vi "disdrometer_output.vi"(0 "Filepath":path, 5 "Data Array":string[](array[string]), 7 "Timestamp":dbl, 9 "Format String":string[](array[string])=["000", "001", "002"], 11 "Error In":errorcluster) -> (15 "Error Out":errorcluster)   [LabVIEW 2018]
doc: "Creates or appends a line to a text file at Filepath, adding the data in Data Array. Appends the Timestamp to the front of the line, and formats the array with tabs between each element."
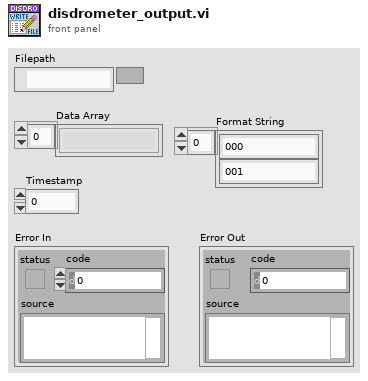
[diagram p1: front panel]
types:
  T1 = enum16{"open", "replace", "create", "open or create", "replace or create", "replace or create with confirmation"}
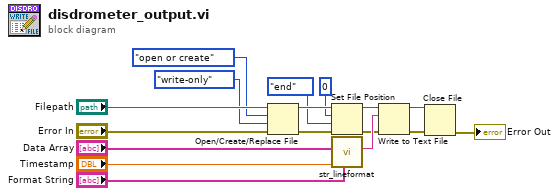
[diagram p0: block diagram]
diagram:
  n1 = Open/Create/Replace File(file path (use dialog)="Filepath", error in="Error In", operation (0:open)=T1."open or create", access (0:read/write)=enum16{"read/write", "read-only", "write-only"}."write-only") -> (refnum out=w11:refnum<file>, error out=w10:errorcluster)  [unwired: 3 out]
  n2 = Set File Position(offset (in bytes) (0)=i64 0, refnum=w11, from (0:start)=enum16{"start", "end", "current"}."end", error in=w10) -> (refnum out=w8:refnum<file>, error out=w9:errorcluster)
  n3 = call "str_lineformat.vi"("Format String"="Format String", "Timestamp"="Timestamp", "String Array"="Data Array") -> ("Formatted String"=w15:string)  [unwired: 8 in]
  n4 = Write to Text File(file (use dialog)=w8, text=w15, error in=w9) -> (refnum out=w5:refnum<file>, error out=w4:errorcluster)  [unwired: 1 in, 1 out]
  n5 = Close File(refnum=w5, error in=w4) -> (error out=→"Error Out":errorcluster)  [unwired: 1 out]
